vi "calculateuncertainty.vi"(0 "refractive index, real":sgl=1.3 step=0.01 format="%.3f", 1 "refractive index, imaginary":sgl=0.1 step=0.01 format="%.3f", 2 "Extinction ExtinctionUncertainity Size parameter and Number ofS sizes 2":T1={"Extinction"=[], "Extinction Uncertainty"=[], "Size parameters"=[], "Number ofSizes"=0.0, "GeometricCrossSection"=[], "Wave Length"=0.0, "SMPS Sizes"=[], "Concentration"=[], "Double Charge Correction"=FALSE, "Extincation Factor"=1.0, "Diameter Factor"=1.0, "Diameter Offset"=0.0, "Extinction Factor Flag"=FALSE, "Diameter Factor Flag"=FALSE, "Diameter Offset Flag"=FALSE, "Sizes"=[], "ExtinctionOrAbsorptionOrScattering"=0} {"ExtinctionOrAbsorptionOrScattering" scale=0.0..2.0}) -> (3 "Real Part (one retrieval)":dbl format="%_4g", 4 "Uncertainty in Real part":dbl format="%#_1g", 5 "Imaginary part (one retrieval)":dbl format="%.3f", 6 "Uncertainty in Imaginary part":dbl format="%#_1g")   [LabVIEW 2011]
uses:
  BaesDataTypeDefinition.ctl
  <vilib>/Analysis/1siggen.llb/Ramp Pattern by Samples.vi
  <vilib>/Analysis/NI_AALBase.lvlib
panel:
  out "Chi Squared Imaginary":dbl[](array[numeric])=[1.7458156608733746, 2.259167774761544, 3.8146805575036473, 6.411304839763114, 10.047860655679122, 14.723114992903353, 20.436242940217376, 27.185713979953526, 34.970304890261, 43.78954822493611, 53.641277932357234]
  out "Ramp Pattern Imaginary":dbl[](array[numeric])=[0.1567711018030022, 0.1577711018030022, 0.1587711018030022, 0.1597711018030022, 0.1607711018030022, 0.1617711018030022, 0.1627711018030022, 0.1637711018030022, 0.1647711018030022, 0.1657711018030022, 0.1667711018030022]
  out "Chi Squared Real Part":dbl[](array[numeric])=[1.7458156608733746, 1.8138021473076842, 2.0074981029054553, 2.3266971611922957, 2.7715418766952578, 3.341681604102128, 4.037207690645187, 4.858019718358637, 5.804017563211861, 6.875028835060166, 8.070943802271257]
  out "Ramp Pattern":dbl[](array[numeric])=[1.6300546159031506, 1.6310546159031505, 1.6320546159031506, 1.6330546159031507, 1.6340546159031506, 1.6350546159031505, 1.6360546159031506, 1.6370546159031507, 1.6380546159031506, 1.6390546159031505, 1.6400546159031506]
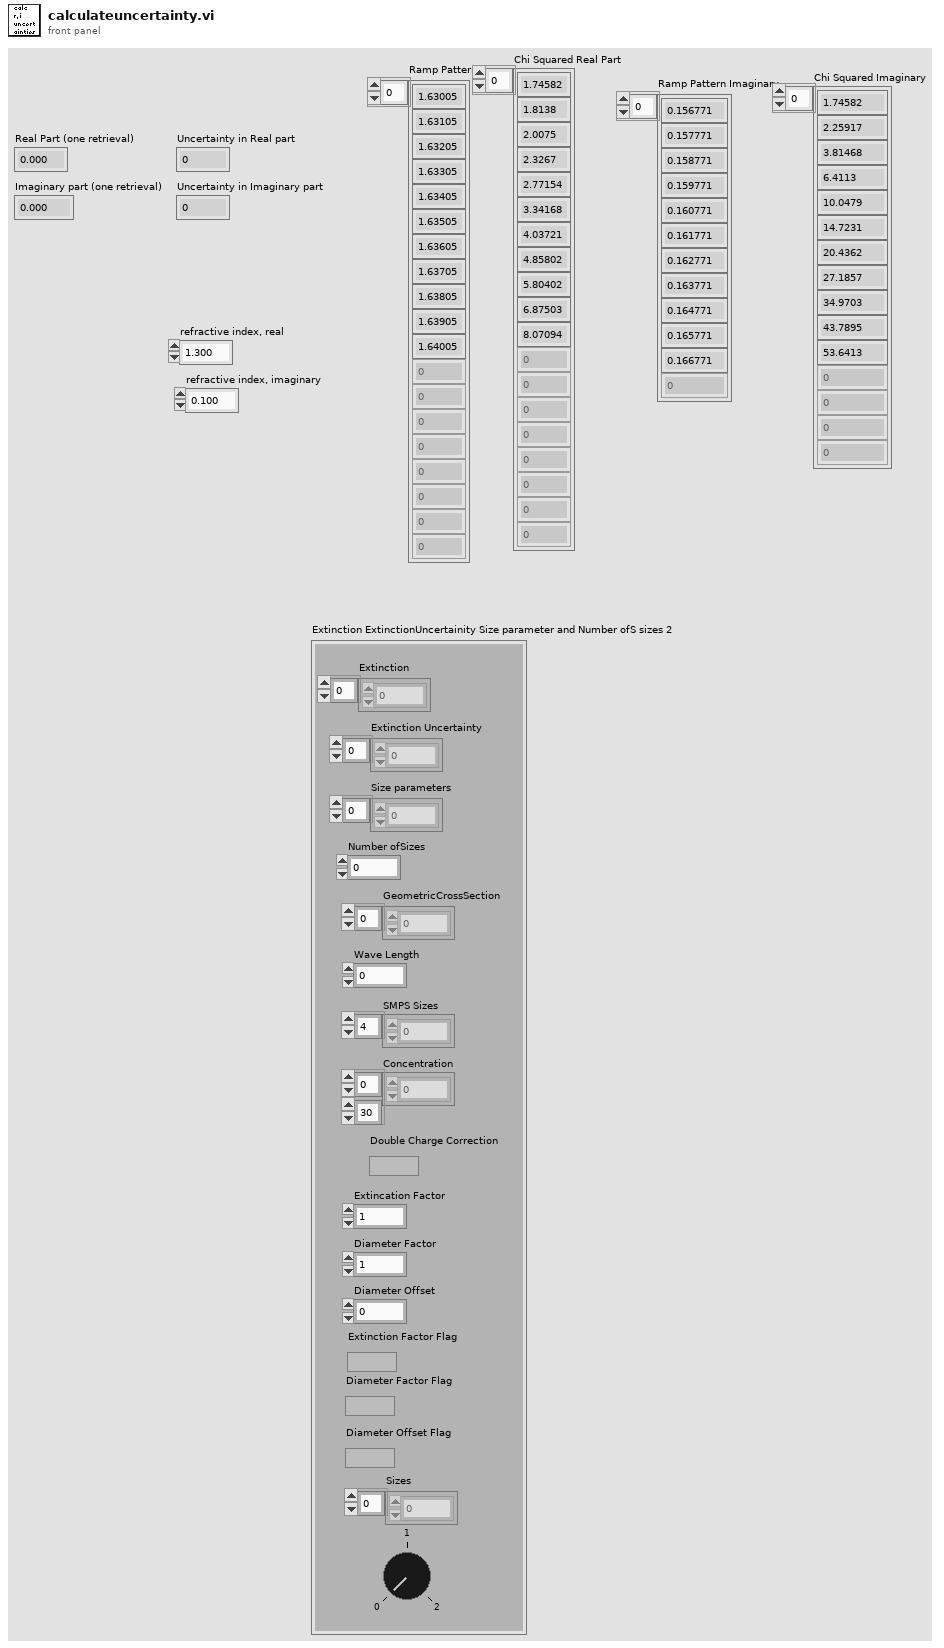
[diagram p1: front panel]
types:
  T1 = typedef "BaesDataTypeDefinition.ctl" = cluster{"Extinction":dbl[], "Extinction Uncertainty":dbl[], "Size parameters":dbl[], "Number ofSizes":dbl, "GeometricCrossSection":dbl[], "Wave Length":dbl, "SMPS Sizes":dbl[], "Concentration":dbl[][], "Double Charge Correction":bool, "Extincation Factor":dbl, "Diameter Factor":dbl, "Diameter Offset":dbl, "Extinction Factor Flag":bool, "Diameter Factor Flag":bool, "Diameter Offset Flag":bool, "Sizes":dbl[], "ExtinctionOrAbsorptionOrScattering":i8}
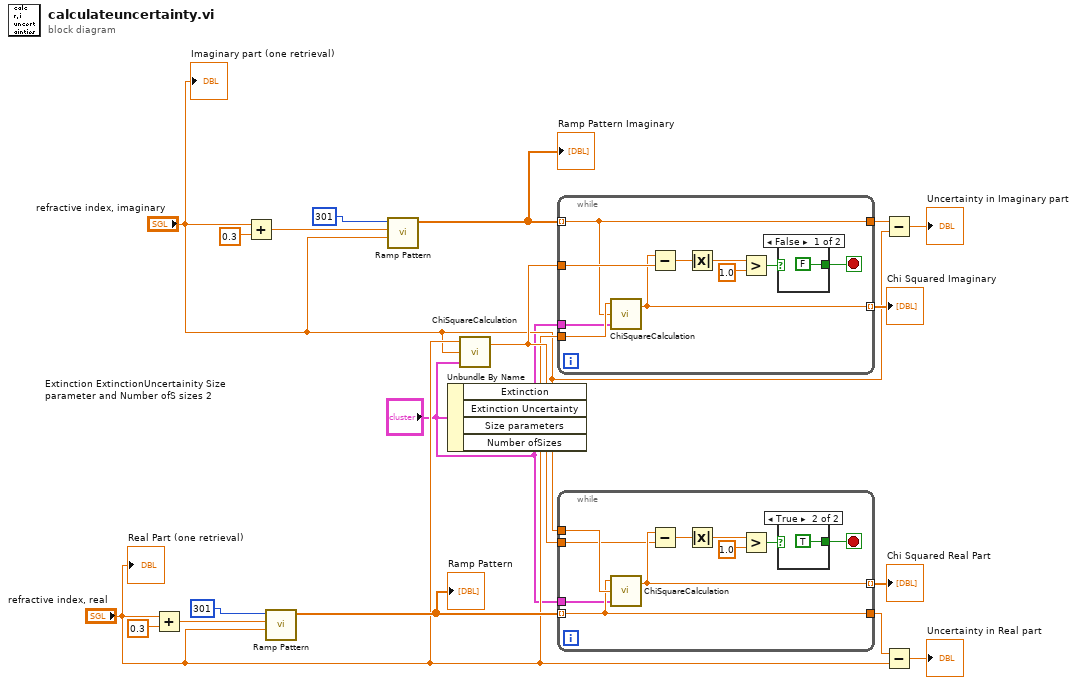
[diagram p0: block diagram]
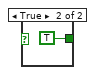
[diagram p2: hidden frame]
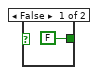
[diagram p3: hidden frame]
diagram:
  n1 = Add(x="refractive index, real", y=0.3) -> (x+y=w17:dbl)
  n2 = Add(x="refractive index, imaginary", y=0.3) -> (x+y=w12:dbl)
  n3 = call-poly <vilib>:"Ramp Pattern.vi"("start"="refractive index, real", "end"=w17, "samples"=301) -> ("Ramp Pattern"=w15:dbl[])  [unwired: 7 in, 1 out]
  "Ramp Pattern" <- w15
  n4 = call-poly <vilib>:"Ramp Pattern.vi"("start"="refractive index, imaginary", "end"=w12, "samples"=301) -> ("Ramp Pattern"=w10:dbl[])  [unwired: 7 in, 1 out]
  "Ramp Pattern Imaginary" <- w10
  n5 = Unbundle By Name("Extinction ExtinctionUncertainity Size parameter and Number ofS sizes 2") -> ()  [unwired: 4 out]
  n6 = call "ChiSquareCalculation.vi"("Extinction ExtinctionUncertainity Size parameter and Number ofS sizes 2"="Extinction ExtinctionUncertainity Size parameter and Number ofS sizes 2", "refractive index, imaginary"="refractive index, imaginary", "refractive index, real"="refractive index, real") -> ("Chi Squared"=w4:dbl)  [unwired: 1 out]
  n7 = while {
    tunnel: w10 -> [w20] mode=indexing
    tunnel: [w22] -> w9 mode=indexing
    tunnel: "refractive index, real" -> [w21]
    tunnel: w4 -> [w23]
    tunnel: [w20] -> w6
    tunnel: "Extinction ExtinctionUncertainity Size parameter and Number ofS sizes 2" -> [w19]
    stop <- w24 stop-if-true
    n8 = call "ChiSquareCalculation.vi"("Extinction ExtinctionUncertainity Size parameter and Number ofS sizes 2"=w19, "refractive index, imaginary"=w20, "refractive index, real"=w21) -> ("Chi Squared"=w22:dbl)  [unwired: 1 out]
    n9 = Subtract(x=w22, y=w23) -> (x-y=w28:dbl)
    n10 = Absolute Value(x=w28) -> (abs(x)=w27:dbl)
    n11 = Greater?(x=w27, y=1.0) -> (0:w25:bool)
    n12 = case shown="False" w25 {
      tunnel: [FALSE TRUE] -> w24
      frame False {
      }
      frame True {
      }
    }
  }
  "Chi Squared Imaginary" <- w9
  n13 = while {
    tunnel: w15 -> [w32] mode=indexing
    tunnel: "refractive index, imaginary" -> [w40]
    tunnel: [w39] -> w14 mode=indexing
    tunnel: w4 -> [w38]
    tunnel: [w32] -> w8
    tunnel: "Extinction ExtinctionUncertainity Size parameter and Number ofS sizes 2" -> [w31]
    stop <- w33 stop-if-true
    n14 = call "ChiSquareCalculation.vi"("Extinction ExtinctionUncertainity Size parameter and Number ofS sizes 2"=w31, "refractive index, imaginary"=w40, "refractive index, real"=w32) -> ("Chi Squared"=w39:dbl)  [unwired: 1 out]
    n15 = Subtract(x=w39, y=w38) -> (x-y=w37:dbl)
    n16 = Absolute Value(x=w37) -> (abs(x)=w36:dbl)
    n17 = Greater?(x=w36, y=1.0) -> (0:w34:bool)
    n18 = case shown="True" w34 {
      tunnel: [FALSE TRUE] -> w33
      frame False {
      }
      frame True {
      }
    }
  }
  "Chi Squared Real Part" <- w14
  n19 = Subtract(x=w6, y="refractive index, imaginary") -> (x-y=→"Uncertainty in Imaginary part":dbl)
  n20 = Subtract(x=w8, y="refractive index, real") -> (x-y=→"Uncertainty in Real part":dbl)
  "Real Part (one retrieval)" <- "refractive index, real"
  "Imaginary part (one retrieval)" <- "refractive index, imaginary"
